vi "DialogBox_oneButton_General_UIvi.vi"(6 "show close button?":bool, 7 "Button Name":string, 8 "error in (no error)":errorcluster, 9 "Blink?":bool, 10 "Message in":string, 11 "Dialogbox header":string) -> (0 "error out":errorcluster, 3 "Proceed?":bool)   [LabVIEW 2015, in "ZenGage v3.0 UI.lvclass"]
uses:
  ZenGage v3.0 UI.lvclass
panel:
  in  "cancel":bool
  out "Dialog Box out":string
  in  "OK button":bool
  out "Message display":string
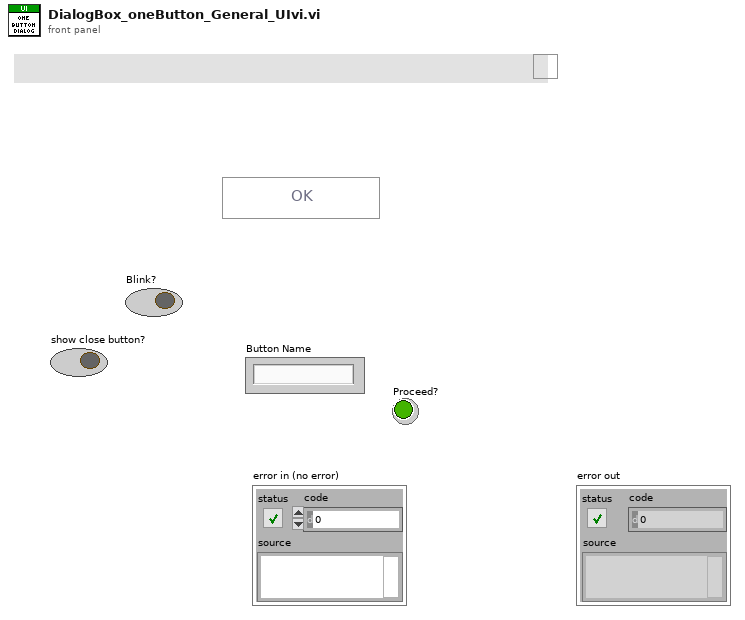
[diagram p1: front panel]
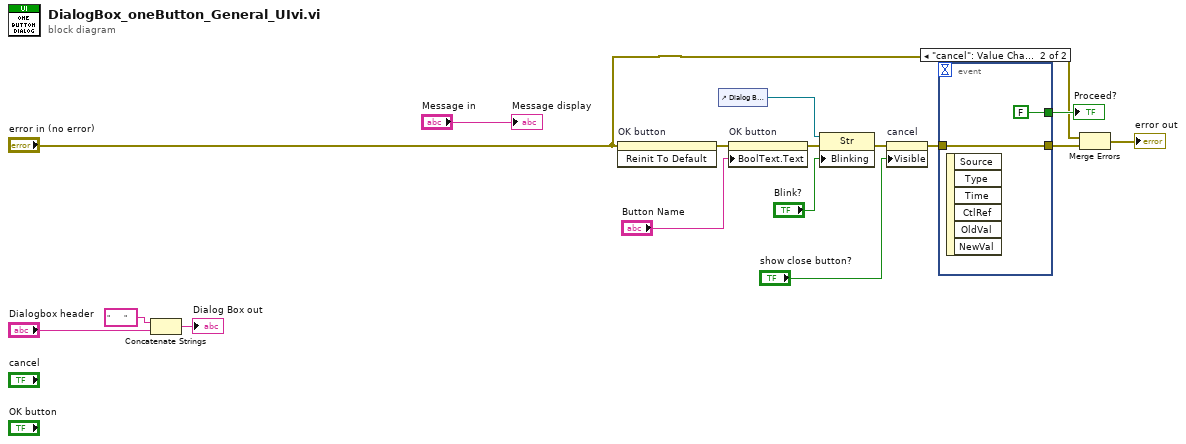
[diagram p0: block diagram]
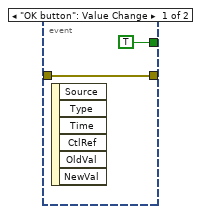
[diagram p2: hidden frame]
diagram:
  n1 = Concatenate Strings("       " ("string"), "Dialogbox header") -> (→"Dialog Box out":string)
  n2 = invoke on="OK button" class="Bool (strict)" method="Reinit To Default"(error in="error in (no error)") -> (error out=w6:errorcluster)  [unwired: 2 in, 2 out]
  n3 = control-ref of="Dialog Box out"() -> (w14:refnum<vi>)
  n4 = property on="OK button" class="Bool (strict)"(error in=w6, "BoolText.Text"="Button Name") -> (error out=w5:errorcluster)  [unwired: 1 in, 1 out]
  n5 = property class="Str"(reference=w14, error in=w5, "Blinking"="Blink?") -> (error out=w10:errorcluster)  [unwired: 1 out]
  n6 = property on="cancel" class="Bool"(error in=w10, "Visible"="show close button?") -> (error out=w9:errorcluster)  [unwired: 1 in, 1 out]
  n7 = event shown="[1] \"cancel\": Value Change" {
    selector: _ -> [_ _]
    dyn-events: _ -> [_ _]
    timeout: _ -> [_ _]
    tunnel: [TRUE FALSE] -> w16
    tunnel: w9 -> [w17 w19]
    tunnel: [w17 w19] -> w4
    event "OK button": Value Change {
      n8 = event-data() -> ()  [unwired: 1 in, 6 out]
    }
    event "cancel": Value Change {
      n9 = event-data() -> ()  [unwired: 1 in, 6 out]
    }
  }
  "Proceed?" <- w16
  n10 = Merge Errors("error in (no error)", w4) -> (→"error out":errorcluster)
  "Message display" <- "Message in"
